vi "Str2Clust.vi"(4 "error in (no error)":errorcluster, 5 "String":string, 7 "Clust Refnum":refnum<vi>) -> (0 "error out":errorcluster)   [LabVIEW 2010]
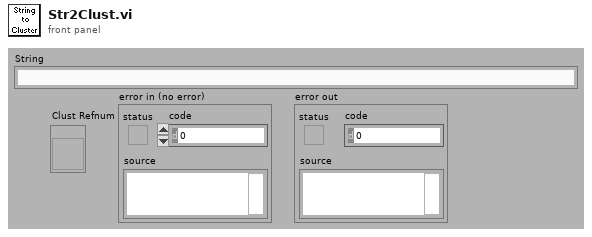
[diagram p1: front panel]
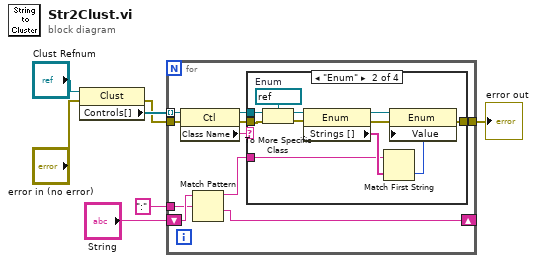
[diagram p0: block diagram]
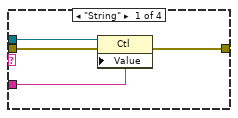
[diagram p2: hidden frame]
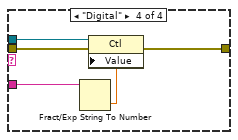
[diagram p4: hidden frame]
diagram:
  n1 = property on="Property Node" class="Clust"(reference="Clust Refnum", error in="error in (no error)") -> (error out=w3:errorcluster, "Controls[]"=w7:refnum<vi>[])  [unwired: 1 out]
  n2 = for {
    tunnel: w7 -> [w17] mode=indexing
    shift-right: [w15] -> _
    shift-left: "String" -> [w14]
    tunnel: ":" ("format string") -> [w12]
    tunnel: w3 -> [w10]
    tunnel: [w8] -> w1
    n3 = property class="Ctl"(reference=w17, error in=w10) -> (reference out=w11:refnum<vi>, error out=w9:errorcluster, "Class Name"=w16:string)
    n4 = Match Pattern(string=w14, regular expression=w12) -> (before substring=w13:string, after substring=w15:string)  [unwired: 1 in, 2 out]
    n5 = case shown="\"Enum\"" w16 {
      tunnel: w11 -> [w21 w31 _ w38]
      tunnel: w13 -> [w20 w28 _ w37]
      tunnel: w9 -> [w19 w25 w33 w35]
      tunnel: [w18 w22 w33 w34] -> w8
      frame "String" {
        n6 = property class="Ctl"(reference=w21, error in=w19, "Value"=w20) -> (error out=w18:errorcluster)  [unwired: 1 out]
      }
      frame "Enum" {
        w32 = refnum<vi> refnum  # Enum
        n7 = To More Specific Class(target class=w32, reference=w31, error in=w25) -> (specific class reference=w30:refnum<vi>, error out=w24:errorcluster)
        n8 = property class="Enum"(reference=w30, error in=w24) -> (reference out=w26:refnum<vi>, error out=w23:errorcluster, "Strings []"=w29:string[])
        n9 = Match First String(2:w29, 3:w28) -> (0:w27:i32)  [unwired: 1 out]
        n10 = property class="Enum"(reference=w26, error in=w23, "Value"=w27) -> (error out=w22:errorcluster)  [unwired: 1 out]
      }
      frame "Any", Default {
      }
      frame "Digital" {
        n11 = Fract/Exp String To Number(string=w37) -> (number=w36:dbl)  [unwired: 3 in, 1 out]
        n12 = property class="Ctl"(reference=w38, error in=w35, "Value"=w36) -> (error out=w34:errorcluster)  [unwired: 1 out]
      }
    }
  }
  "error out" <- w1
